vi "getForceFieldForceSpringyWallsDebounced.vi"(0 "Boundary X coords":dbl[](array[numeric]), 2 "Desired force direction vector":dbl[](array[numeric]), 5 "Boundary Y coords":dbl[](array[numeric]), 7 "Current control point coordinates":dbl[](array[numeric]), 9 "Scaled debounce boundary X coords":dbl[](array[numeric]), 11 "Scaled debounce boundary Y coords":dbl[](array[numeric]), 12 "forceScalingConstantK":dbl) -> (4 "Output FX FY Fz 0 0 0":dbl[](array[numeric]))   [LabVIEW 2017]
uses:
  <vilib>/Analysis/_algsub.llb/Real Vector Norm.vi
  <vilib>/Analysis/_algsub.llb/Complex Vector Norm.vi
  <vilib>/imath/engines/lvmath2/RunTimeEngine/IndexRead/NIMS V(S).vi
  <instcachedir>/0/NIMS V(S)_0488751826AF41519A22953C041130DC.lvgen/NIMS V(S)_0488751826AF41519A22953C041130DC_000.vi
  <vilib>/imath/engines/lvmath2/RunTimeEngine/BuiltInFunctions/is_inpolygon/NIMS_is_inpolygon(V).vi
  <vilib>/imath/engines/lvmath2/RunTimeEngine/ErrorHandling/NIMS_Create Error From Enums.vi
  <vilib>/imath/engines/lvmath2/RunTimeSupport/NIMS_Get Scalar_w Error.vi
  <instcachedir>/0/NIMS_Get Scalar_w Error_1987D997E87247DDAC16EA23A5E9E4FC.lvgen/NIMS_Get Scalar_w Error_1987D997E87247DDAC16EA23A5E9E4FC_010.vi
  <vilib>/imathl/engines/lvmath/Functions/Error Handling/Create Error.vi
  LabVIEW Data/MathScriptVIs/MCStatic_38590875332_a85215386faa3ccbe6a0cf488bf2b96b.vi
  <instcachedir>/0/MCStatic_38590875332_a85215386faa3ccbe6a0cf488bf2b96b_687210BDAE424B85ACC6A4EA1761F058.lvgen/MCStatic_38590875332_a85215386faa3ccbe6a0cf488bf2b96b_687210BDAE424B85ACC6A4EA1761F058_000.vi
  <vilib>/imath/engines/lvmath2/RunTimeEngine/NodeEndStatement/NIMS_NodeEndStatement_Output.vi
  <instcachedir>/0/NIMS_NodeEndStatement_Output_53EC0D466D134D7ABD903AC30B43404B.lvgen/NIMS_NodeEndStatement_Output_53EC0D466D134D7ABD903AC30B43404B_009.vi
  <vilib>/imath/engines/lvmath2/RunTimeEngine/ErrorHandling/NIMS_Finalize Error.vi
  LabVIEW Data/projectPointOnto2DPolygon.m
  <vilib>/Analysis/NI_AALPro.lvlib
panel:
  in  "DebounceAreaForceConstant":dbl
  out "Computed F magnitude":dbl
  out "Distance current pos to center pos":dbl
  # "Inputs"
  # "Key parameters set in this subVI"
  # "Outputs"
  # "Other values"
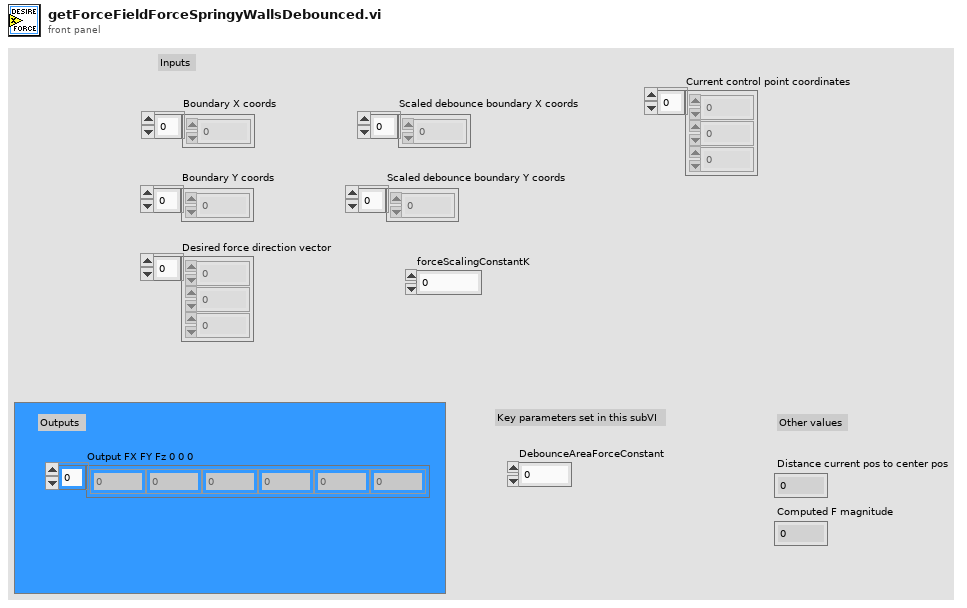
[diagram p1: front panel]
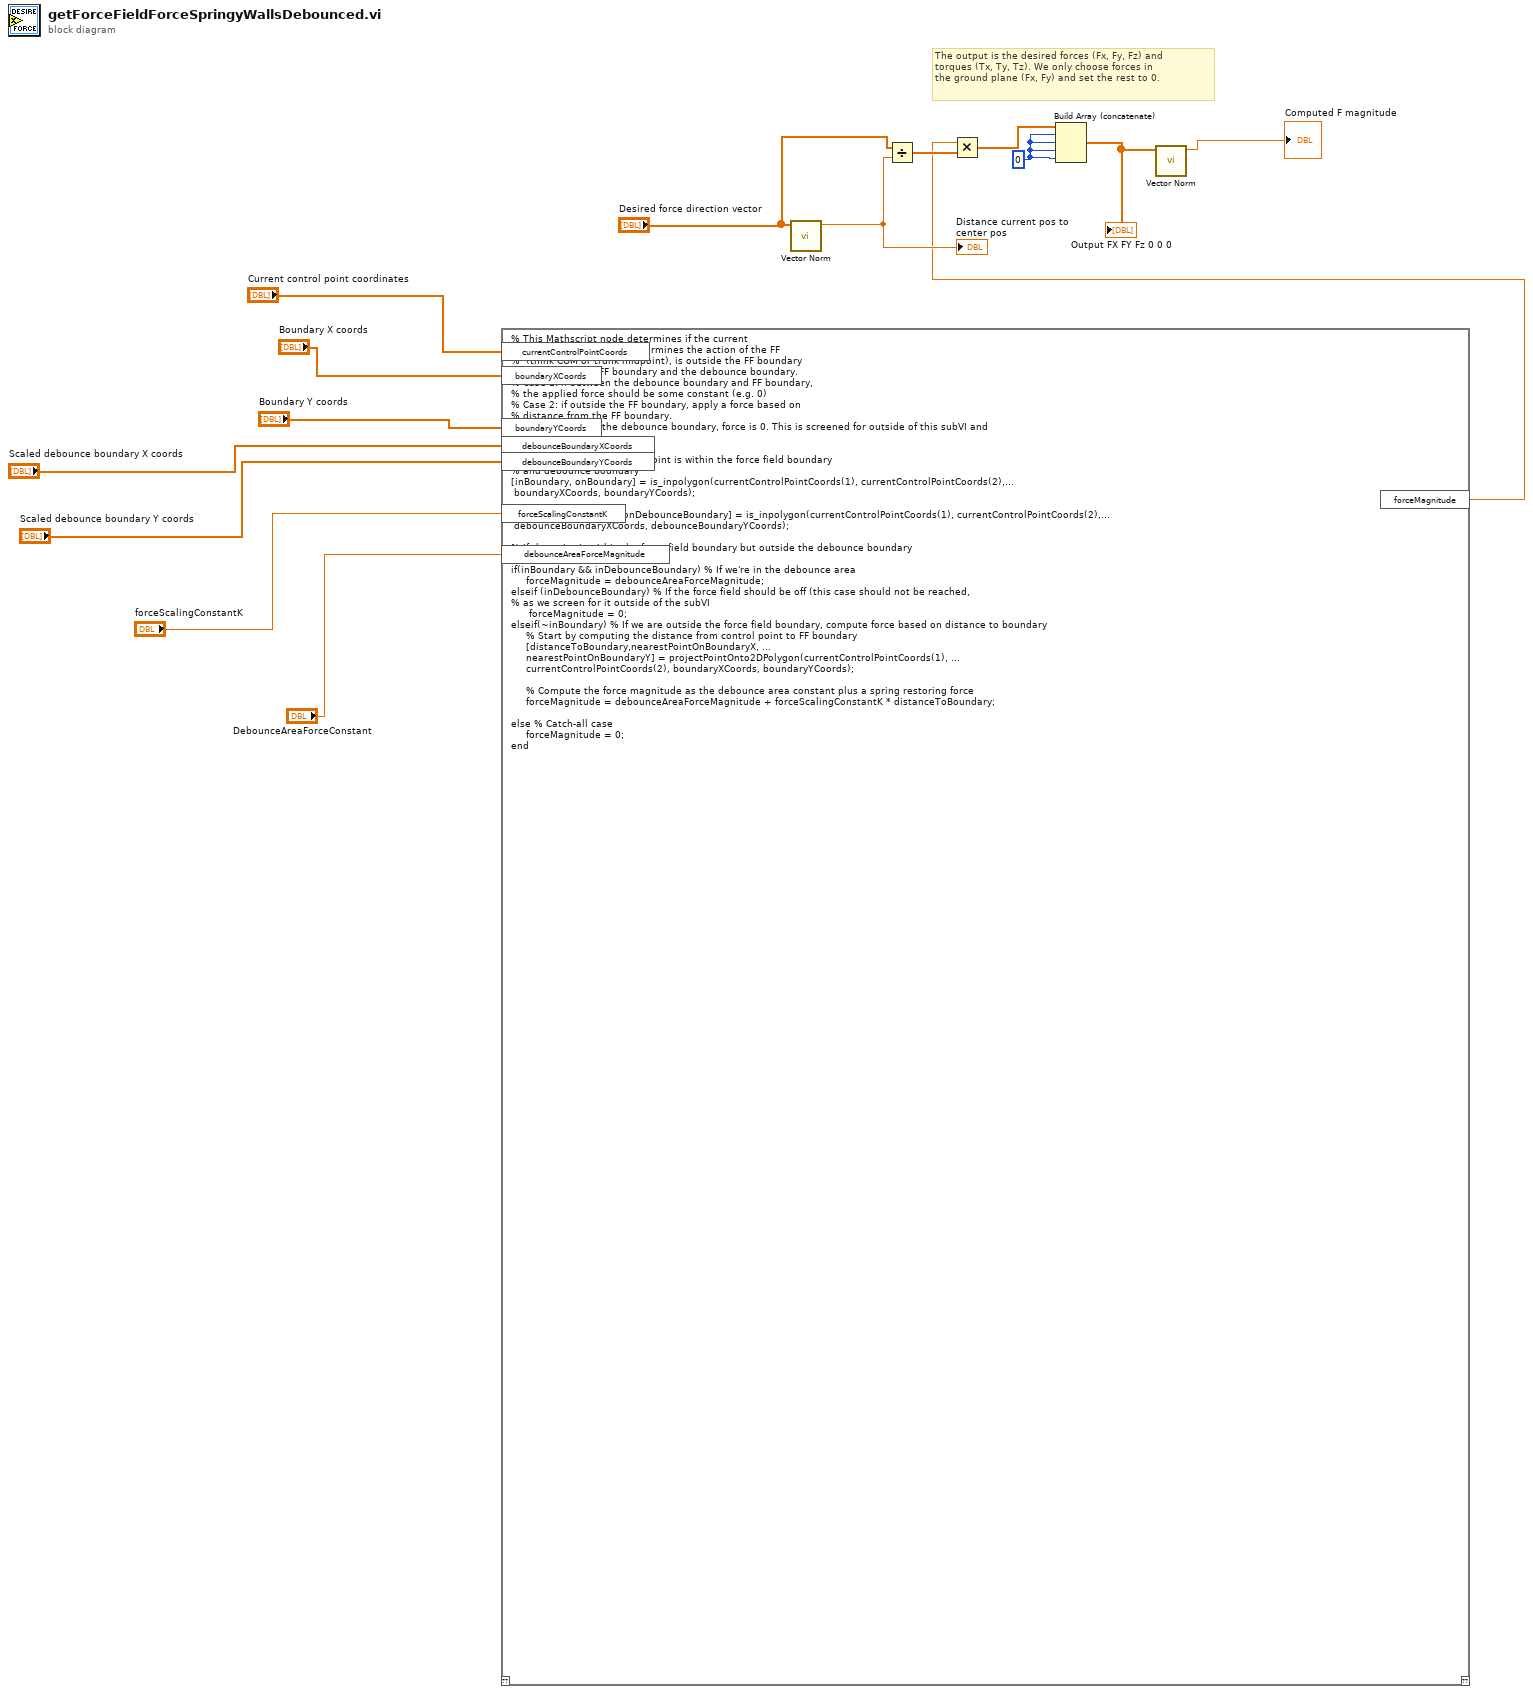
[diagram p0: block diagram]
diagram:
  w1 = 0
  # "The output is the desired forces (Fx, Fy, Fz) and \ntorques (Tx, Ty, Tz). We only choose forces in \nthe ground plane (Fx, Fy) and set the rest to 0."
  n1 = mathscript code="% This Mathscript node determines if the current\n% \"control point,\" which determines the action of the FF\n%  (think COM or trunk midpoint), is outside the FF boundary\n% or between the FF boundary and the debounce boundary. \n% Case 1: if between the debounce boundary and FF boundary, \n% the applied force should be some constant (e.g. 0)\n% Case 2: if outside the FF boundary, apply a force based on \n% distance from the FF boundary.\n% Case 3: if inside the debounce boundary, force is 0. This is screened for outside of this subVI and \n% should not occur.\n\n% Start by computing if the point is within the force field boundary\n% and debounce boundary\n[inBoundary, onBoundary] = is_inpolygon(currentControlPointCoords(1), currentControlPointCoords(2),...\n boundaryXCoords, boundaryYCoords);\n\n[inDebounceBoundary, onDebounceBoundary] = is_inpolygon(currentControlPointCoords(1), currentControlPointCoords(2),...\n debounceBoundaryXCoords, debounceBoundaryYCoords);\n\n% If the point is within the force field boundary but outside the debounce boundary\nforceMagnitude = 0;\nif(inBoundary && inDebounceBoundary) % If we're in the debounce area\n     forceMagnitude = debounceAreaForceMagnitude;\nelseif (inDebounceBoundary) % If the force field should be off (this case should not be reached,\n% as we screen for it outside of the subVI\n      forceMagnitude = 0;\nelseif(~inBoundary) % If we are outside the force field boundary, compute force based on distance to boundary\n     % Start by computing the distance from control point to FF boundary \n     [distanceToBoundary,nearestPointOnBoundaryX, ...\n     nearestPointOnBoundaryY] = projectPointOnto2DPolygon(currentControlPointCoords(1), ...\n     currentControlPointCoords(2), boundaryXCoords, boundaryYCoords);\n\n     % Compute the force magnitude as the debounce area constant plus a spring restoring force\n     forceMagnitude = debounceAreaForceMagnitude + forceScalingConstantK * distanceToBoundary;\n\nelse % Catch-all case\n     forceMagnitude = 0;\nend"("boundaryXCoords"="Boundary X coords", "boundaryYCoords"="Boundary Y coords", "debounceBoundaryXCoords"="Scaled debounce boundary X coords", "debounceBoundaryYCoords"="Scaled debounce boundary Y coords", "currentControlPointCoords"="Current control point coordinates", "forceScalingConstantK"="forceScalingConstantK", "debounceAreaForceMagnitude"="DebounceAreaForceConstant") -> ("forceMagnitude"=w2:cdb)  [unwired: 1 in, 1 out]
  n2 = call-poly <vilib>:"Vector Norm.vi"("Input Vector"="Desired force direction vector") -> ("norm"=w14:dbl)  [unwired: 9 in, 1 out]
  "Distance current pos to center pos" <- w14
  n3 = Divide(x="Desired force direction vector", y=w14) -> (x/y=w15:dbl[])
  n4 = Multiply(x=w2, y=w15) -> (x*y=w13:cdb[])
  n5 = Build Array (concatenate)(w13, w1, w1, w1, w1) -> (w12:cdb[])
  "Output FX FY Fz 0 0 0" <- w12
  n6 = call-poly <vilib>:"Vector Norm.vi"("Input Vector"=w12) -> ("norm"=→"Computed F magnitude":dbl)  [unwired: 9 in, 1 out]
